vi "Build Tree.vi"(5 "Panel":refnum<vi>, 7 "Tree":refnum<vi>, 9 "Changed Actors":refnum<class "Message Enqueuer.lvclass">[](array[class]), 10 "Monitor Data":refnum<class "Monitor Data.lvclass">) -> (2 "Stopped Actors":string[](array[string]))   [LabVIEW 2017, in "MGI-Monitored Actor.lvlib" / "Classic Monitor.lvclass"]
doc: "Manages the tree.\n\nCopyright: MGI 2016\nAuthor: Derek Trepanier"
uses:
  Classic Monitor.lvclass
  monitored-actor-core/Source/Monitor Data/Monitor Data.lvclass
  <vilib>/ActorFramework/Message Enqueuer/Message Enqueuer.lvclass
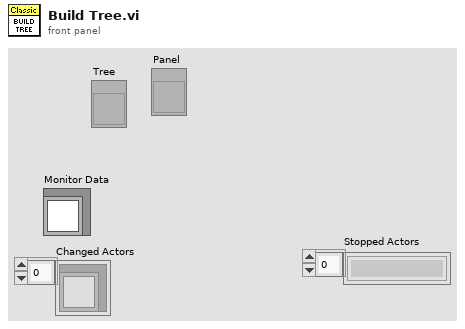
[diagram p1: front panel]
types:
  T1 = typedef "MGI-Monitored Actor Core.lvlib/Monitor Data.lvclass/Actor Data.ctl" = cluster{"Actor Type":string, "Actor Cores":string[], "Self":refnum<class "Message Enqueuer.lvclass">, "Caller":refnum<class "Message Enqueuer.lvclass">, "Actor Label":string, "Last Ping":dbl}
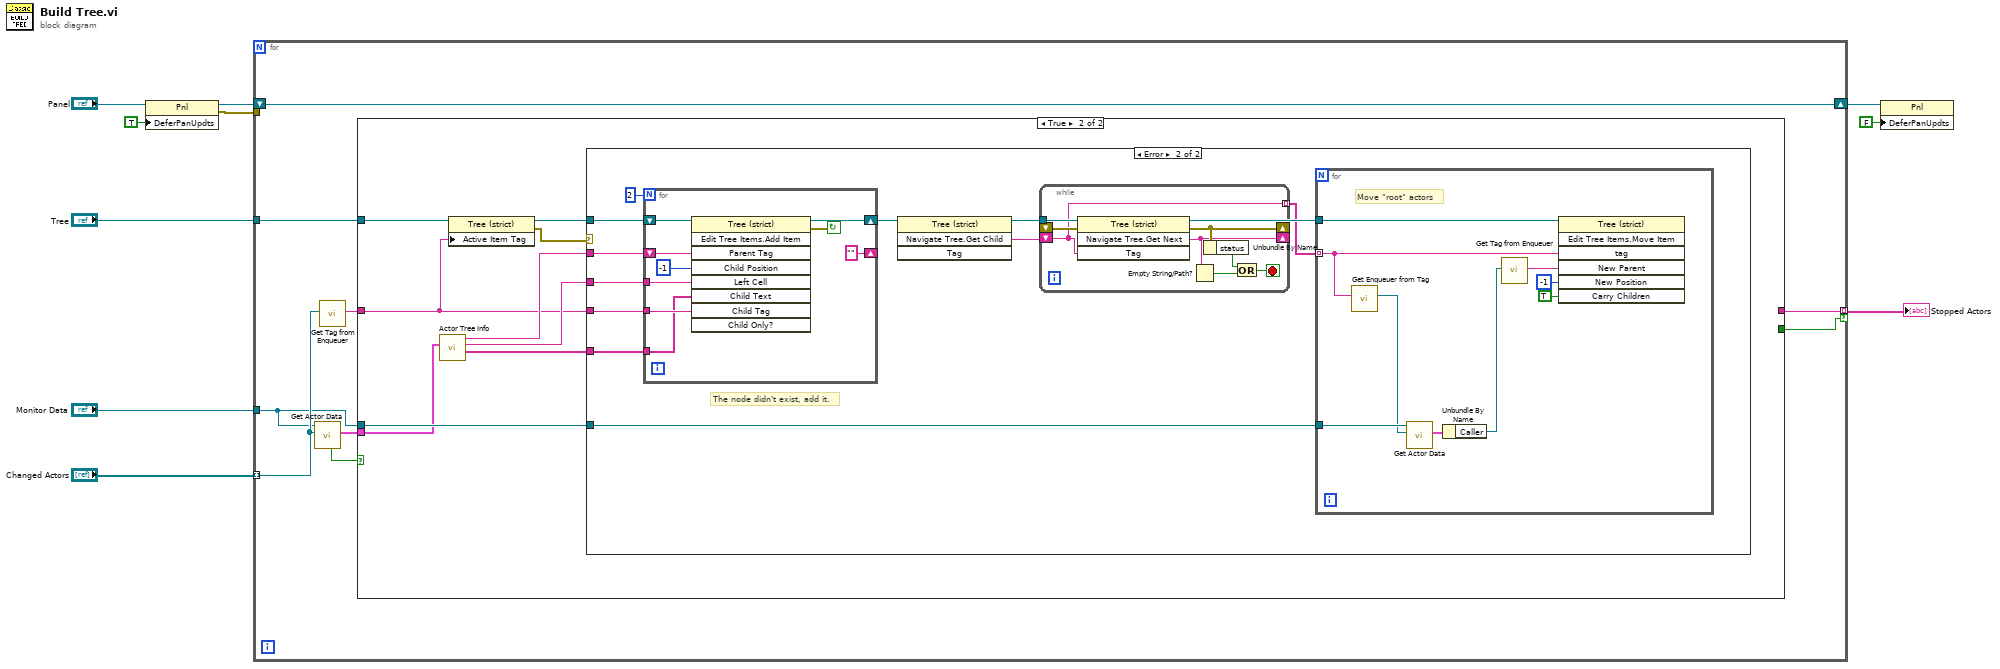
[diagram p0: block diagram]
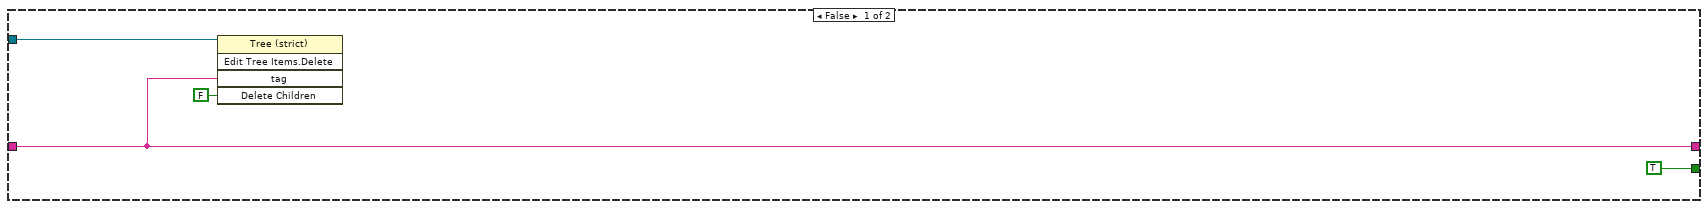
[diagram p2: hidden frame]
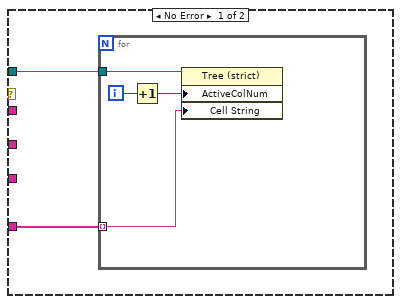
[diagram p3: hidden frame]
diagram:
  n1 = property class="Pnl"(reference="Panel", "DeferPanUpdts"=TRUE ("Defer Panel Updates")) -> (reference out=w5:refnum<vi>, error out=w1:errorcluster)  [unwired: 1 in]
  n2 = for {
    tunnel: "Monitor Data" -> [w11]
    tunnel: "Tree" -> [w19]
    shift-right: [w18] -> w4
    shift-left: w5 -> [w18]
    tunnel: "Changed Actors" -> [w16] mode=indexing
    tunnel: [w13] -> w2 mode=indexing if=w12
    tunnel: w1 -> [_]
    n3 = call "Get Actor Data.vi"("Actor's Self Q"=w16, "Monitor Data in"=w11) -> ("Actor Data"=w17:T1, "Found?"=w14:bool)  [unwired: 6 in, 2 out]
    n4 = call "Get Tag from Enqueuer.vi"("Enqueuer"=w16) -> ("Tag"=w15:string)  [unwired: 10 in]
    n5 = case shown="True" w14 {
      tunnel: w19 -> [w23 w32]
      tunnel: w11 -> [_ w27]
      tunnel: w17 -> [_ w26]
      tunnel: w15 -> [w21 w24]
      tunnel: [w21 _] -> w13
      tunnel: [TRUE _] -> w12
      frame False {
        n6 = invoke class="Tree (strict)" method="Edit Tree Items.Delete"(reference=w23, "tag"=w21, "Delete Children"=FALSE ("Delete Children?")) -> ()  [unwired: 2 in, 5 out]
      }
      frame True {
        n7 = call "Actor Tree Info.vi"("Actor Data"=w26) -> ("Column Data"=w29:string[], "Node Name"=w25:string, "Parent Tag"=w28:string)  [unwired: 8 in]
        n8 = property class="Tree (strict)"(reference=w32, "Active Item Tag"=w24) -> (reference out=w30:refnum<vi>, error out=w31:errorcluster)  [unwired: 1 in]
        n9 = case shown="Error" w31 {
          tunnel: w30 -> [w34 w49]
          tunnel: w29 -> [w33 w48]
          tunnel: w28 -> [_ w47]
          tunnel: w27 -> [_ w45]
          tunnel: w25 -> [_ w44]
          tunnel: w24 -> [_ w43]
          frame No Error {
            n10 = for {
              tunnel: w34 -> [w38]
              tunnel: w33 -> [w36] mode=indexing
              i -> [w37]
              n11 = Increment(x=w37) -> (x+1=w35:i32)
              n12 = property class="Tree (strict)"(reference=w38, "ActiveColNum"=w35, "Cell String"=w36) -> ()  [unwired: 1 in, 2 out]
            }
          }
          frame Error {
            # "The node didn't exist, add it."
            n13 = for {
              N: 2 -> [_]
              tunnel: w48 -> [w58]
              shift-right: ["" ("Parent Tag")] -> _
              shift-left: w47 -> [w64]
              shift-right: [w61] -> w42
              shift-left: w49 -> [w66]
              tunnel: w44 -> [w60]
              tunnel: w43 -> [w59]
              stop <- w62 continue-if-true
              n14 = invoke class="Tree (strict)" method="Edit Tree Items.Add Item"(reference=w66, "Parent Tag"=w64, "Child Position"=-1, "Left Cell"=w60, "Child Text"=w58, "Child Tag"=w59) -> (reference out=w61:refnum<vi>, error out=w62:errorcluster)  [unwired: 3 in, 7 out]
            }
            n15 = invoke class="Tree (strict)" method="Navigate Tree.Get Child"(reference=w42) -> (reference out=w41:refnum<vi>, "Navigate Tree:Get Child"=w40:string)  [unwired: 3 in, 2 out]
            n16 = while {
              shift-right: [w51] -> _
              shift-left: w40 -> [w50]
              tunnel: w41 -> [w57]
              shift-right: [w52] -> _
              shift-left: _ -> [w56]
              tunnel: [w50] -> w39 mode=indexing
              stop <- w54 stop-if-true
              n17 = invoke class="Tree (strict)" method="Navigate Tree.Get Next"(reference=w57, error in=w56, "Tag"=w50) -> (error out=w52:errorcluster, "Navigate Tree:Get Next Item"=w51:string)  [unwired: 1 in, 2 out]
              n18 = Empty String/Path?(string/path=w51) -> (empty?=w55:bool)
              n19 = Unbundle By Name(w52) -> ("status"=w53:bool)
              n20 = Compound Arithmetic op=OR(w53, w55) -> (w54:bool)
            }
            n21 = for {
              tunnel: w45 -> [w75]
              tunnel: w41 -> [w72]
              tunnel: w39 -> [w67] mode=indexing
              # "Move \"root\" actors"
              n22 = call "Get Enqueuer from Tag.vi"("Tag"=w67) -> ("Enqueuer"=w74:refnum<class "Message Enqueuer.lvclass">)  [unwired: 10 in]
              n23 = call "Get Actor Data.vi"("Actor's Self Q"=w74, "Monitor Data in"=w75) -> ("Actor Data"=w73:T1)  [unwired: 6 in, 3 out]
              n24 = Unbundle By Name(w73) -> ("Caller"=w71:refnum<class "Message Enqueuer.lvclass">)
              n25 = call "Get Tag from Enqueuer.vi"("Enqueuer"=w71) -> ("Tag"=w70:string)  [unwired: 10 in]
              n26 = invoke class="Tree (strict)" method="Edit Tree Items.Move Item"(reference=w72, "tag"=w67, "New Parent"=w70, "New Position"=-1, "Carry Children"=TRUE ("Carry Children?")) -> ()  [unwired: 2 in, 7 out]
            }
          }
        }
      }
    }
  }
  "Stopped Actors" <- w2
  n27 = property class="Pnl"(reference=w4, "DeferPanUpdts"=FALSE ("Defer Panel Updates")) -> ()  [unwired: 1 in, 2 out]
